vi "calculo de f_k.vi"(11 "iteração":dbl) -> (3 "F_k":T1)   [LabVIEW 2018]
uses:
  <vilib>/Analysis/Matrix/Datatypes/RealMatrix.ctl
  <vilib>/Analysis/Matrix/NI_Matrix.lvlib
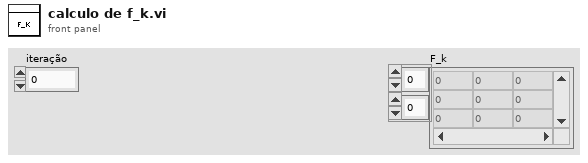
[diagram p1: front panel]
types:
  T1 = typedef "NI_Matrix.lvlib/RealMatrix.ctl" = dbl[][]
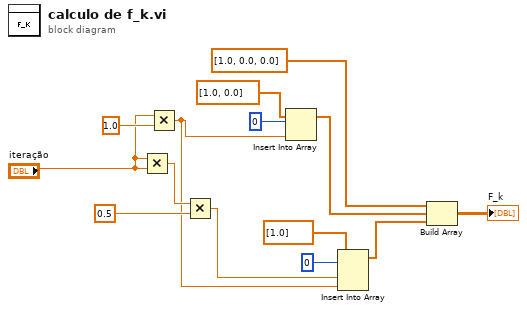
[diagram p0: block diagram]
diagram:
  n1 = Multiply(x="iteração", y="iteração") -> (x*y=w6:dbl)
  n2 = Multiply(x="iteração", y=1.0) -> (x*y=w5:dbl)
  n3 = Multiply(x=w6, y=0.5) -> (x*y=w4:dbl)
  n4 = Insert Into Array(array=dbl[] [1.0, 0.0] ("element"), index=0, new element=w5) -> (w11:dbl[])
  n5 = Insert Into Array(array=dbl[] [1.0], index=0, new element #1=w4, new element #2=w5) -> (w3:dbl[])
  n6 = Build Array(dbl[] [1.0, 0.0, 0.0] ("element"), w11, w3) -> (→"F_k":T1)
